vi "teste 3456A.vi"() -> ()   [LabVIEW 2018]
uses:
  <vilib>/Instr/_visa.llb/GPIB Status Boolean Array.ctl
panel:
  out "ibsta":T1
  in  "error in (no error)":errorcluster
  out "error out":errorcluster
  in  "stop 2":bool
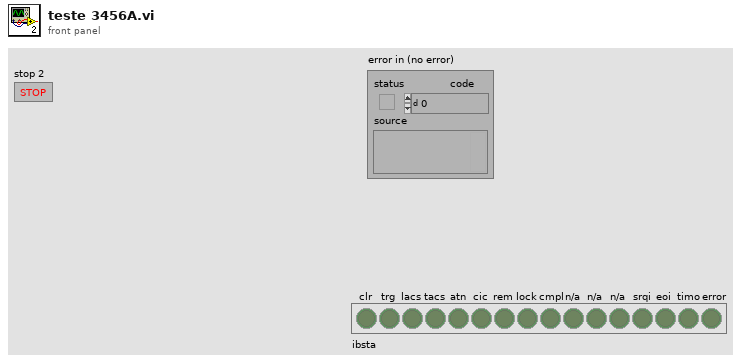
[diagram p1: front panel]
types:
  T1 = typedef "GPIB Status Boolean Array.ctl" = bool[]
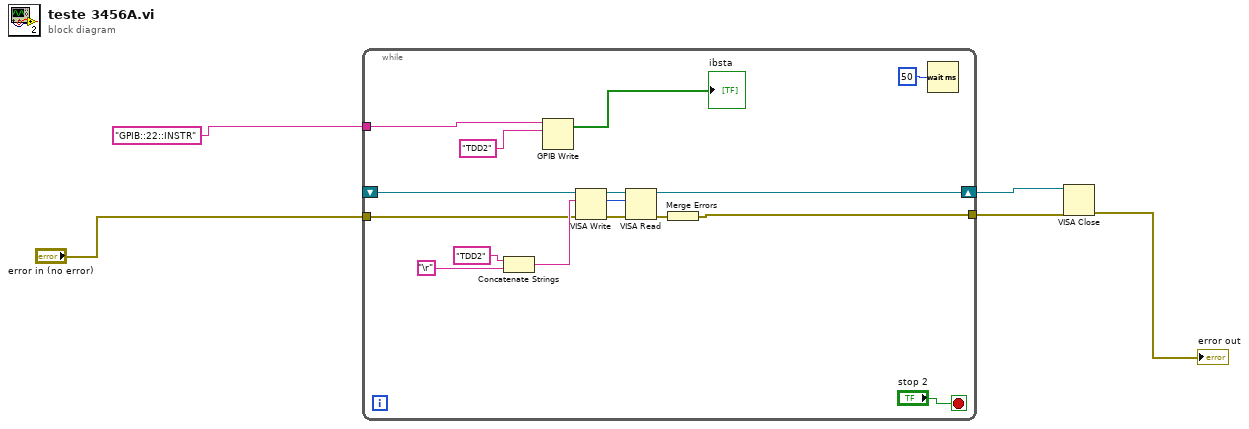
[diagram p0: block diagram]
diagram:
  n1 = while {
    tunnel: [w13] -> w4
    shift-right: [w12] -> w5
    shift-left: _ -> [w14]
    tunnel: "error in (no error)" -> [w9]
    tunnel: "GPIB::22::INSTR" ("address string") -> [w7]
    stop <- "stop 2" stop-if-true
    n2 = Concatenate Strings("TDD2" ("string"), "\r") -> (w17:string)
    n3 = GPIB Write(0:w7, 1:"TDD2" ("string")) -> (5:→"ibsta":bool[])  [unwired: 3 in, 1 out]
    n4 = VISA Write(VISA resource name=w14, write buffer=w17, error in (no error)=w9) -> (VISA resource name out=w18:refnum<visa-resource-name>, return count=w20:u32, error out=w21:errorcluster)
    n5 = VISA Read(VISA resource name=w18, byte count=w20, error in (no error)=w21) -> (VISA resource name out=w12:refnum<visa-resource-name>, error out=w19:errorcluster)  [unwired: 2 out]
    n6 = Merge Errors(w19) -> (w13:errorcluster)
    n7 = Wait (ms)(milliseconds to wait=u32 50) -> ()  [unwired: 1 out]
  }
  n8 = VISA Close(VISA resource name=w5, error in (no error)=w4) -> (error out=→"error out":errorcluster)
